vi "New_Magazine_Execute.vi"() -> ()   [LabVIEW 2019]
uses:
  Utility_VIs/Basic_Motor_Modes.ctl
  <vilib>/Rock Robotics/WPI/Solenoid/WPI_SolenoidValue.ctl
  New_Magazine_Globals.vi
  Sensing/Sensor_Values.vi
panel:
  in  "Spin_Up_Threshold(RPM)":dbl
  in  "Spinup_Speed":dbl
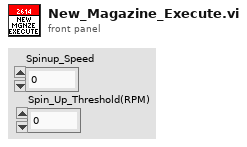
[diagram p1: front panel]
types:
  T1 = typedef "Basic_Motor_Modes.ctl" = enum16{"Percent_Voltage", "Speed_Control", "Position_Control", "Current"}
  T2 = typedef "WPI_SolenoidValue.ctl" = enum16{"Off", "On", "Forward", "Reverse"}
  T3 = typedef "New_Magazine_Cluster.ctl" = cluster{"Control_States":T4, "Firing":bool, "Throttle":dbl, "Spinning Up":bool, "Off":bool, "Extend_Magazine_Manual":bool}
  T4 = typedef "New_Magazine_Control_States.ctl" = enum16{"No-Op", "Up", "Down", "Manual", "Fire", "Spinning Up"}
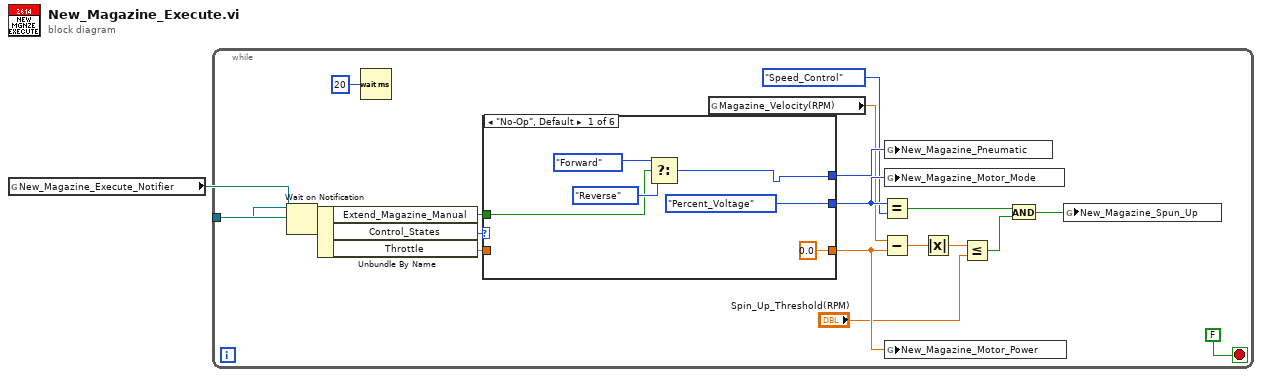
[diagram p0: block diagram]
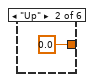
[diagram p2: hidden frame]
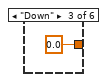
[diagram p3: hidden frame]
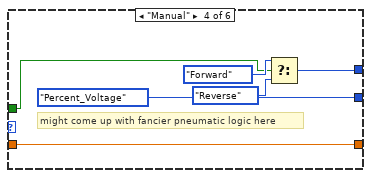
[diagram p4: hidden frame]
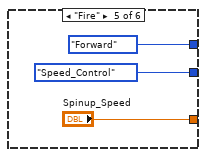
[diagram p5: hidden frame]
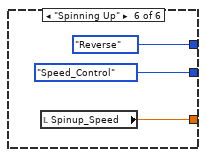
[diagram p6: hidden frame]
diagram:
  n1 = global read "New_Magazine_Globals.vi" "New_Magazine_Execute_Notifier"() -> (w1:refnum<notifier>)
  n2 = while {
    tunnel: w1 -> [w17]
    stop <- FALSE stop-if-true
    n3 = Wait on Notification(notifier=w17) -> (notification=w16:T3)  [unwired: 3 in, 3 out]
    n4 = Unbundle By Name(w16) -> ("Extend_Magazine_Manual"=w2:bool, "Control_States"=w15:T4, "Throttle"=w13:dbl)
    n5 = Wait (ms)(milliseconds to wait=u32 20 ("millisecond timer value")) -> ()  [unwired: 1 out]
    n6 = case shown="\"No-Op\", Default" w15 {
      tunnel: [0.0 ("New_Magazine_Motor_Power") 0.0 ("New_Magazine_Motor_Power") 0.0 ("New_Magazine_Motor_Power") w33 "Spinup_Speed" w39] -> w8
      tunnel: [w20 _ _ w31 WPI_SolenoidValue."Forward" ("New_Magazine_Pneumatic") WPI_SolenoidValue."Reverse" ("New_Magazine_Pneumatic")] -> w14
      tunnel: [Basic_Motor_Modes."Percent_Voltage" ("New_Magazine_Motor_Mode") _ _ Basic_Motor_Modes."Percent_Voltage" ("New_Magazine_Motor_Mode") Basic_Motor_Modes."Speed_Control" ("New_Magazine_Motor_Mode") Basic_Motor_Modes."Speed_Control" ("New_Magazine_Motor_Mode")] -> w12
      tunnel: w13 -> [_ _ _ w33 _ _]
      tunnel: w2 -> [w21 _ _ w28 _ _]
      frame "No-Op", Default {
        n7 = Select(t=WPI_SolenoidValue."Forward" ("New_Magazine_Pneumatic"), s=w21, f=WPI_SolenoidValue."Reverse" ("New_Magazine_Pneumatic")) -> (s? t:f=w20:T2)
      }
      frame "Up" {
      }
      frame "Down" {
      }
      frame "Manual" {
        # "might come up with fancier pneumatic logic here"
        n8 = Select(t=WPI_SolenoidValue."Forward" ("New_Magazine_Pneumatic"), s=w28, f=WPI_SolenoidValue."Reverse" ("New_Magazine_Pneumatic")) -> (s? t:f=w31:T2)
      }
      frame "Fire" {
      }
      frame "Spinning Up" {
        n9 = local read "Spinup_Speed"() -> (w39:dbl)
      }
    }
    n10 = global read "Sensor_Values.vi" "Magazine_Velocity(RPM)"() -> (w9:dbl)
    n11 = Equal?(x=w12, y=Basic_Motor_Modes."Speed_Control") -> (x = y?=w10:bool)
    n12 = Subtract(x=w9, y=w8) -> (x-y=w6:dbl)
    n13 = global write "New_Magazine_Globals.vi" "New_Magazine_Pneumatic"(w14) -> ()
    n14 = global write "New_Magazine_Globals.vi" "New_Magazine_Motor_Mode"(w12) -> ()
    n15 = global write "New_Magazine_Globals.vi" "New_Magazine_Motor_Power"(w8) -> ()
    n16 = Absolute Value(x=w6) -> (abs(x)=w5:dbl)
    n17 = Less Or Equal?(x=w5, y="Spin_Up_Threshold(RPM)") -> (x <= y?=w7:bool)
    n18 = And(x=w10, y=w7) -> (x .and. y?=w3:bool)
    n19 = global write "New_Magazine_Globals.vi" "New_Magazine_Spun_Up"(w3) -> ()
  }
